vi "Test App Adding Process Triggers Broadcast.vi"(8 "error in (no error)":errorcluster, 11 "Rig Test in":refnum<class "Application Dev Test.lvclass">) -> (0 "error out":errorcluster, 3 "Rig Test out":refnum<class "Application Dev Test.lvclass">)   [LabVIEW 2020, in "Application Dev Test.lvclass"]
uses:
  Application Dev Test.lvclass
  C:/Program Files (x86)/National Instruments/LabVIEW 2020/vi.lib/Astemes/LUnit/Test Case.lvclass
  source/Framework/Process/Process.lvclass
  source/Framework/Process/Process.lvclass/Process.ctl
  source/Framework/Application/Application.lvclass/Application.ctl
  <vilib>/Astemes/LUnit/Test Case.lvclass/Test Case.ctl
  <vilib>/Astemes/LUnit/LUnit Assertion Result.lvclass/LUnit Assertion Result.ctl
  <vilib>/Astemes/LUnit/LUnit Test Case Result.lvclass/LUnit Test Case Result.ctl
  <vilib>/Astemes/LUnit/LUnit Method Result.lvclass/LUnit Method Result.ctl
  10a4d3f2-41cc-4c69-b9c3-b472845d1909.vi
  source/Framework/Process/Public/Lifecycle/Get Lifecycle State.vi
  source/Framework/Application/Private/Add Process to Map.vi
  source/Framework/Application/Private/Start Idle Processes if Running.vi
  source/Framework/Application/Private/Throw Error If Process Already in App.vi
  source/Framework/Process/Protected/Messaging/Enqueue Message.vi
  source/Framework/Process/Protected/SubVIs/Set Context.vi
  source/Framework/Broadcast Event Helpers/Execution timer.vi
  <vilib>/Astemes/LUnit/Palette/Pass.vi
  <vilib>/Astemes/LUnit/Palette/Fail.vi
  <vilib>/Astemes/LUnit/Compare Variants.vi
  <vilib>/Astemes/LUnit/Describe Comparison.vi
  <vilib>/Astemes/LUnit/Set Assertion Type.vi
  source/Framework/Process/Private/SubVIs/Wait for finish.vi
  source/Framework/Process/Private/SubVIs/Set Lifecycle State.vi
  <vilib>/Utility/error.llb/Clear Errors.vi
  source/Framework/Application/Public/Get Process.vi
  source/Framework/Process/Private/SubVIs/Handle Debug Data.vi
  source/Framework/Process/Public/Lifecycle/Leave Process Loop.vi
  <vilib>/Astemes/LUnit/Add test result.vi
  <vilib>/Astemes/LUnit/LUnit Write Passed.vi
  <vilib>/Astemes/LUnit/LUnit Write Message.vi
  <vilib>/Astemes/LUnit/LUnit Write Description.vi
  <vilib>/Astemes/LUnit/Variant to string.vi
  <vilib>/Astemes/LUnit/LUnit Write Assertion Type.vi
  source/Framework/Application/Private/Retrieve Process from App.vi
  source/Framework/Application/Private/Parse Process Name.vi
  source/Framework/Application/Private/Get Process from Map.vi
  source/Framework/Logging/Log Debug.vi
  <vilib>/AdvancedString/1D String Array to Delimited String.vi
  <vilib>/Utility/High Resolution Relative Seconds.vi
  <vilib>/Astemes/LUnit/LUnit Record Assertion Result.vi
  source/Framework/Process/Protected/Messaging/Request Message.vi
  <vilib>/AdvancedString/Delimited String to 1D String Array.vi
  <vilib>/Astemes/LUnit/LUnit Aggregate Assertion Results.vi
  source/Framework/Process/Private/SubVIs/Enqueue Request Message.vi
  <vilib>/Astemes/LUnit/Assertion Result/LUnit Read Status.vi
  <vilib>/Astemes/LUnit/LUnit Read Message.vi
  <vilib>/Astemes/LUnit/LUnit Read Description.vi
  <vilib>/Astemes/LUnit/Method Result/LUnit Merge Status.vi
  <vilib>/Astemes/LUnit/LUnit Concatenate result strings.vi
  source/Framework/Application/Application.lvclass
  C:/Git/astemes-triarc-framework/source/Framework/Process/Process.lvclass
  <vilib>/Utility/error.llb/Error Cluster From Error Code.vi
  source/Framework/Process/Private/SubVIs/Wait for Response Message.vi
  source/Framework/Broadcast Event Helpers/Dequeue Broadcast Message.vi
  <vilib>/Utility/Data Type/Get Type Information.vi
  <vilib>/Utility/LVClass/Get LV Class Name.vi
  <vilib>/Astemes/LUnit/LUnit Assertion Result.lvclass
  source/Framework/Broadcast Event Helpers/Broadcast Event Helpers.lvlib
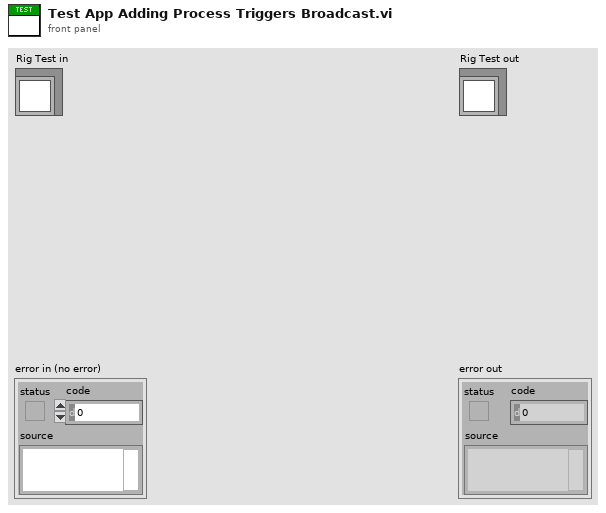
[diagram p1: front panel]
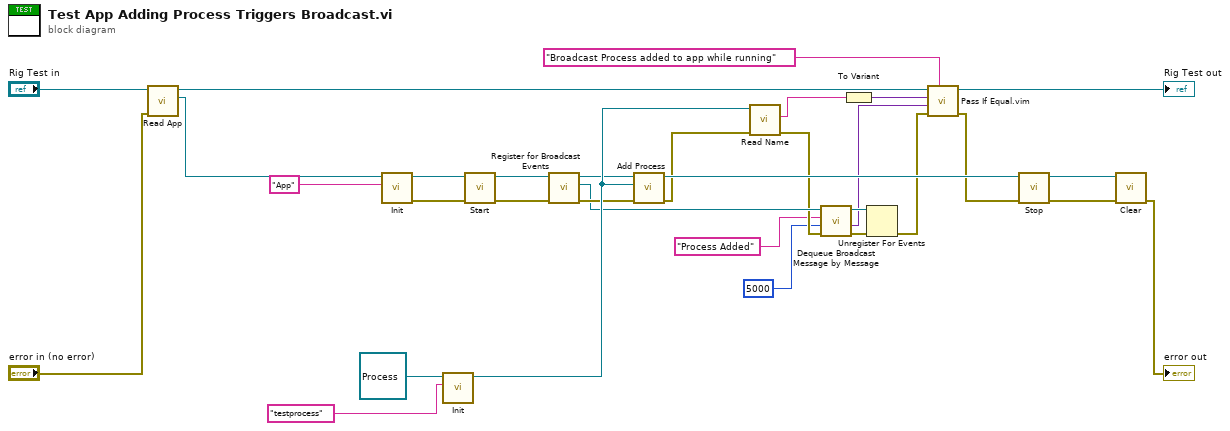
[diagram p0: block diagram]
diagram:
  n1 = call "Read App.vi"("error in (no error)"="error in (no error)", "Application Test In"="Rig Test in") -> ("App out"=w31:refnum<class "Application.lvclass">, "Application Test Out"=w20:refnum<class "Application Dev Test.lvclass">)  [unwired: 7 in, 1 out]
  n2 = call-dynamic "Init.vi"("Name"="App", "Process In"=w31) -> ("error out"=w21:errorcluster, "Process Out"=w22:refnum<class "Application.lvclass">)  [unwired: 8 in]
  n3 = call-dynamic "Init.vi"("Name"="testprocess", "Process In"=refnum<class "Process.lvclass"> refnum ("Process.lvclass")) -> ("Process Out"=w19:refnum<class "Process.lvclass">)  [unwired: 8 in, 1 out]
  n4 = call "Start.vi"("error in (no error)"=w21, "Process In"=w22) -> ("error out"=w23:errorcluster, "Process Out"=w12:refnum<class "Application.lvclass">)  [unwired: 7 in, 1 out]
  n5 = call "Register for Broadcast Events.vi"("error in (no error)"=w23, "Process In"=w12) -> ("error out"=w13:errorcluster, "Event Registration Refnum Out"=w9:refnum<event-registration>, "Process Out"=w11:refnum<class "Application.lvclass">)  [unwired: 7 in]
  n6 = call "Add Process.vi"("error in (no error)"=w13, "Process"=w19, "Application In"=w11) -> ("error out"=w14:errorcluster, "Application Out"=w29:refnum<class "Application.lvclass">)  [unwired: 7 in]
  n7 = call "Read Name.vi"("error in (no error)"=w14, "Process In"=w19) -> ("error out"=w8:errorcluster, "Qualified Name"=w10:string)  [unwired: 6 in, 2 out]
  n8 = call "Dequeue Broadcast Message by Message.vi"("error in (no error)"=w8, "Timeout (-1)"=5000, "Message"="Process Added", "Event Registration Refnum"=w9) -> ("error out"=w7:errorcluster, "Message Data"=w4:variant, "Event Registration Refnum Out"=w5:refnum<event-registration>)  [unwired: 3 in, 2 out]
  n9 = To Variant(anything=w10) -> (Variant=w1:variant)
  n10 = Unregister For Events(event registration refnum=w5, error in=w7) -> (error out=w6:errorcluster)
  n11 = call "Pass If Equal.vim"("Description"="Broadcast Process added to app while running", "error in (no error)"=w6, "Actual"=w4, "Expected"=w1, "LUnit Test Case In"=w20) -> ("error out"=w25:errorcluster, "LUnit Test Case Out"=→"Rig Test out":refnum<class "Application Dev Test.lvclass">)  [unwired: 5 in]
  n12 = call "Stop.vi"("error in (no error)"=w25, "Process In"=w29) -> ("error out"=w17:errorcluster, "Process Out"=w16:refnum<class "Application.lvclass">)  [unwired: 7 in, 1 out]
  n13 = call-dynamic "Clear.vi"("error in (no error)"=w17, "Application In"=w16) -> ("error out"=→"error out":errorcluster)  [unwired: 9 in]
